vi "Signal Acquisition.vi"(0 "Signals Sampling":T4 {"Sample Mode" items=["Finite Samples"=10178, "Continuous Samples"=10123, "Hardware Timed Single Point"=12522]}, 1 "Pressure Signal":T5 {"Terminal Configuration" items=["Default"=-1, "RSE"=10083, "Differential"=10106, "Pseudodifferential"=12529]; "Scale Type" items=["Volts"=10348, "Custom Scale"=10065]}, 2 "Electrode Signals":T1={"Scale Type"=10348, "Terminal Configuration"=10083, "Scale Name"="", "Range [V]"={"max"=10.0, "min"=-10.0}, "Channel 2 [Potential]"="Dev4/ai2", "Channel 1 [Current]"="Dev4/ai2"} {"Terminal Configuration" items=["Default"=-1, "RSE"=10083, "Differential"=10106, "Pseudodifferential"=12529]; "Scale Type" items=["Volts"=10348, "Custom Scale"=10065]}, 5 "error in":errorcluster, 6 "Indicators":T3, 8 "Filter":refnum<vi>, 10 "Filter Led Indicator":refnum<vi>, 12 "IIR filter specifications":refnum<vi>, 13 "Exit":refnum<vi>) -> (19 "error out":errorcluster)   [LabVIEW 2012, in "Signal Acquisition.lvlib"]
uses:
  Signal Acquisition.lvlib
  <vilib>/DAQmx/read.llb/DAQmx Read (Analog 1D Wfm NChan NSamp).vi
  <vilib>/DAQmx/create/channels.llb/DAQmx Create Channel (AI-Voltage-Basic).vi
  <vilib>/DAQmx/configure/timing.llb/DAQmx Timing (Sample Clock).vi
  <vilib>/measure/madcrms.llb/Basic Averaged DC-RMS for 1 Chan.vi
  <vilib>/measure/maspectr.llb/FFT Power Spectrum and PSD for 1 Chan.vi
  <vilib>/DAQmx/miscellaneous.llb/DAQmx Fill In Error Info.vi
  <vilib>/measure/NI_MAPro.lvlib
  <vilib>/measure/macond.llb/IIR Filter for 1 Chan.vi
panel:
  out "Resistance C":dbl
  out "Current":dbl
  out "Resistance":dbl
  out "Pressure":waveform(dbl)
  out "Current Signal":waveform(dbl)
  out "PSD":cluster{"f0":dbl, "df":dbl, "magnitude":dbl[]} {"magnitude" format="%.2p"; "f0" format="%0.2p"; "df" format="%0.2p"}
  out "Filter":bool
  out "Filter Param":T2
  out "Exit":bool
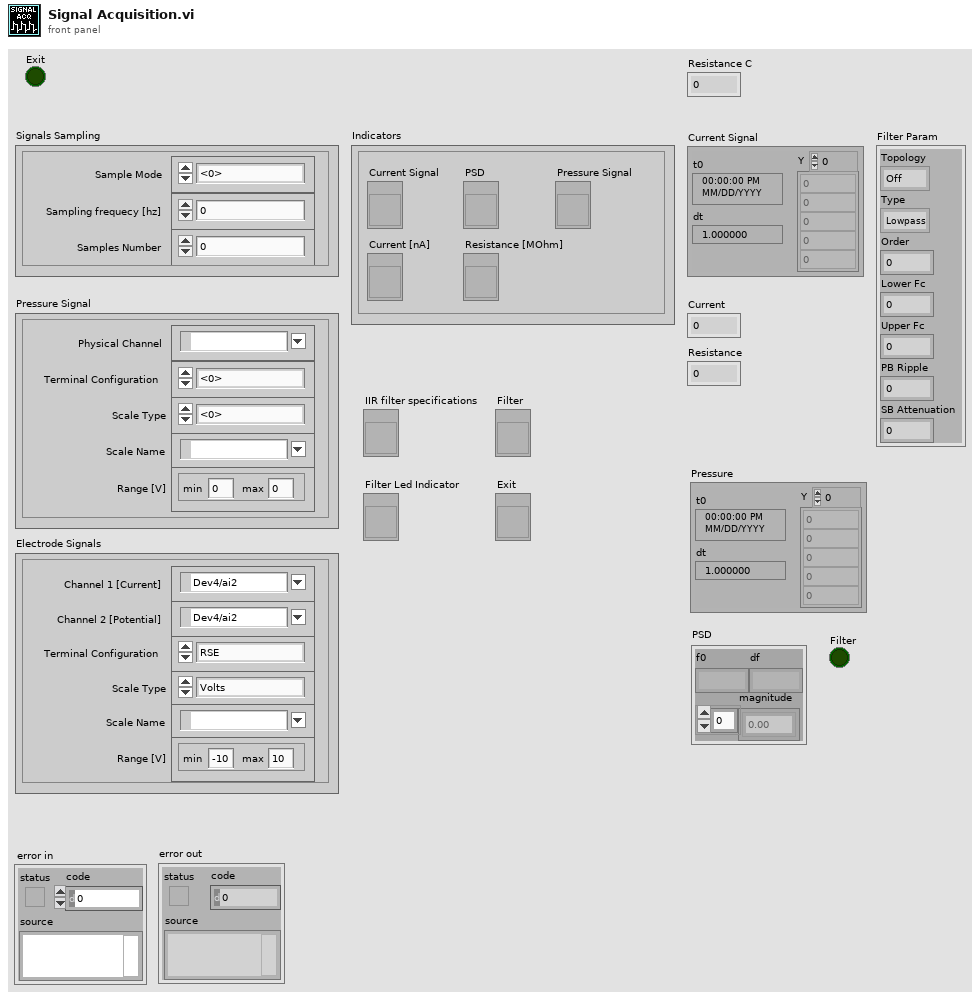
[diagram p1: front panel]
types:
  T1 = cluster{"Scale Type":i32, "Terminal Configuration":i32, "Scale Name":tag, "Range [V]":cluster{"max":dbl, "min":dbl}, "Channel 2 [Potential]":tag, "Channel 1 [Current]":tag}
  T2 = cluster{"Topology":enum16{"Off", "Butterworth", "Chebyshev", "Inverse Chebyshev", "Elliptic", "Bessel"}, "Type":enum16{"Lowpass", "Highpass", "Bandpass", "Bandstop"}, "Order":i32, "Lower Fc":dbl, "Upper Fc":dbl, "PB Ripple":dbl, "SB Attenuation":dbl}
  T3 = cluster{"Current Signal":refnum<vi>, "PSD":refnum<vi>, "Pressure Signal":refnum<vi>, "Current [nA]":refnum<vi>, "Resistance [MOhm]":refnum<vi>}
  T4 = cluster{"Sample Mode":i32, "Sampling frequecy [hz]":dbl, "Samples Number":i32}
  T5 = cluster{"Scale Type":i32, "Terminal Configuration":i32, "Scale Name":tag, "Range [V]":cluster{"max":dbl, "min":dbl}, "Physical Channel":tag}
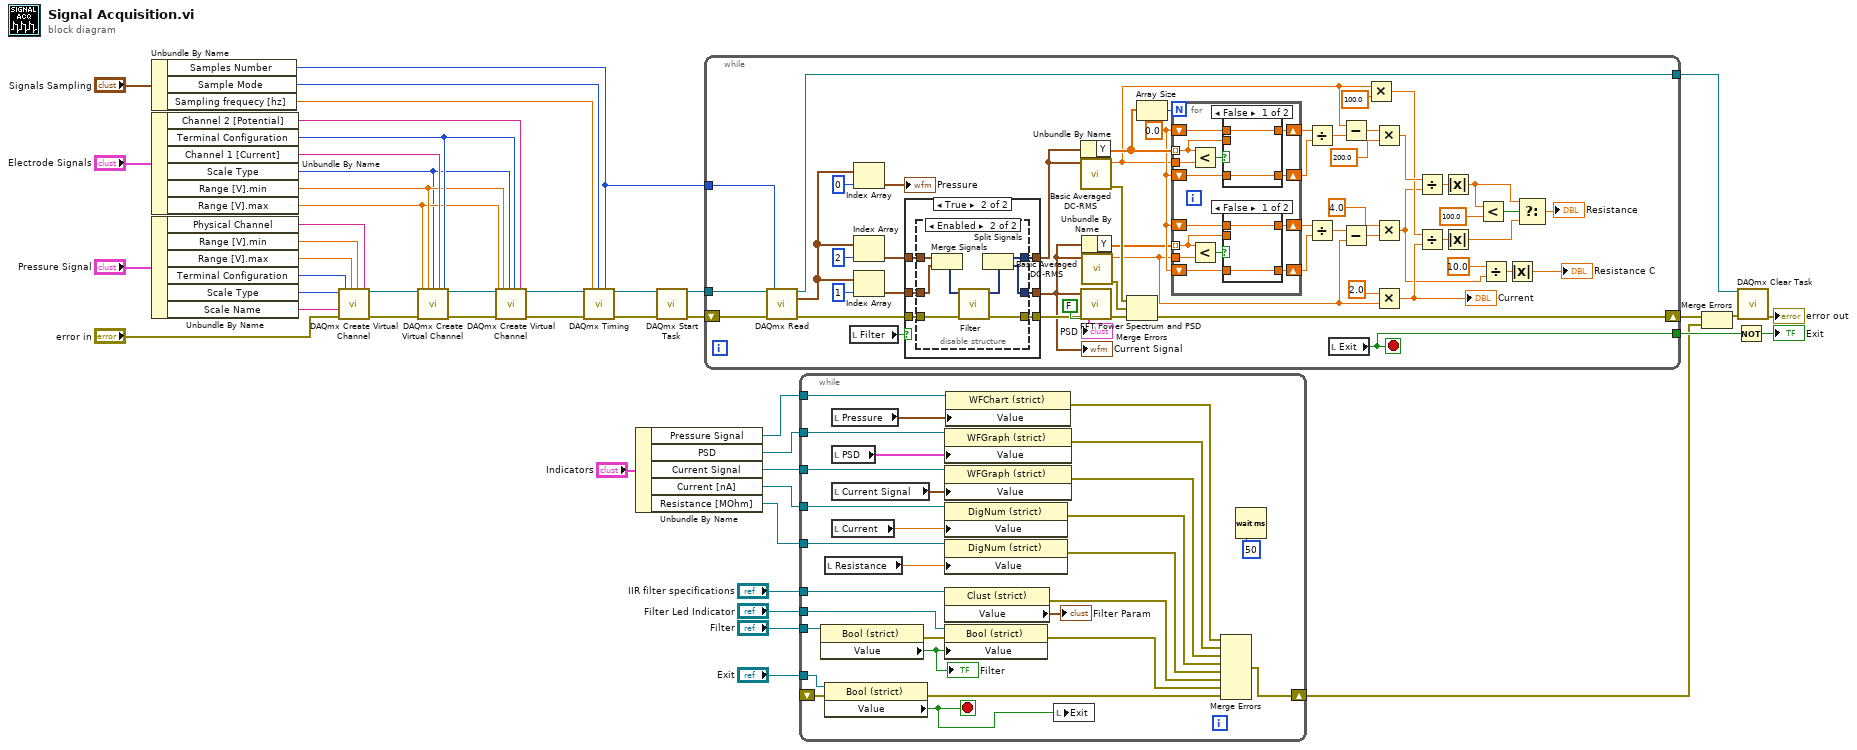
[diagram p0: block diagram]
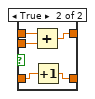
[diagram p2: hidden frame]
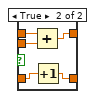
[diagram p3: hidden frame]
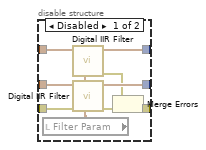
[diagram p5: hidden frame]
diagram:
  n1 = Unbundle By Name("Signals Sampling") -> ("Samples Number"=w26:i32, "Sample Mode"=w25:i32, "Sampling frequecy [hz]"=w24:dbl)
  n2 = Unbundle By Name("Electrode Signals") -> ("Channel 2 [Potential]"=w10:tag, "Terminal Configuration"=w9:i32, "Channel 1 [Current]"=w43:tag, "Scale Type"=w6:i32, "Range [V].min"=w8:dbl, "Range [V].max"=w7:dbl)
  n3 = Unbundle By Name("Pressure Signal") -> ("Physical Channel"=w36:tag, "Range [V].min"=w35:dbl, "Range [V].max"=w34:dbl, "Terminal Configuration"=w33:i32, "Scale Type"=w32:i32, "Scale Name"=w31:tag)
  n4 = call-poly <vilib>:"DAQmx Create Virtual Channel.vi"("maximum value"=w34, "minimum value"=w35, "input terminal configuration"=w33, "physical channels"=w36, "units"=w32, "error in"="error in", "custom scale name"=w31) -> ("task out"=w30:refnum<k21>, "error out"=w29:errorcluster)  [unwired: 7 in]
  n5 = call-poly <vilib>:"DAQmx Create Virtual Channel.vi"("task in"=w30, "maximum value"=w7, "minimum value"=w8, "input terminal configuration"=w9, "physical channels"=w43, "units"=w6, "error in"=w29) -> ("task out"=w11:refnum<k21>, "error out"=w12:errorcluster)  [unwired: 7 in]
  n6 = call-poly <vilib>:"DAQmx Create Virtual Channel.vi"("task in"=w11, "maximum value"=w7, "minimum value"=w8, "input terminal configuration"=w9, "physical channels"=w10, "units"=w6, "error in"=w12) -> ("task out"=w4:refnum<k21>, "error out"=w5:errorcluster)  [unwired: 7 in]
  n7 = call-poly <vilib>:"DAQmx Timing.vi"("task/channels in"=w4, "sample mode"=w25, "samples per channel"=w26, "rate"=w24, "error in"=w5) -> ("task out"=w41:refnum<k21>, "error out"=w42:errorcluster)  [unwired: 9 in]
  n8 = Unbundle By Name("Indicators") -> ("Pressure Signal"=w14:refnum<vi>, "PSD"=w3:refnum<vi>, "Current Signal"=w18:refnum<vi>, "Current [nA]"=w2:refnum<vi>, "Resistance [MOhm]"=w1:refnum<vi>)
  n9 = call <vilib>:"DAQmx Start Task.vi"("task/channels in"=w41, "error in"=w42) -> ("task out"=w39:refnum<k21>, "error out"=w40:errorcluster)  [unwired: 12 out]
  n10 = while {
    tunnel: w39 -> [w101]
    tunnel: w26 -> [w99]
    tunnel: [w98] -> w44
    shift-right: [w66] -> w16
    shift-left: w40 -> [w100]
    tunnel: [w97] -> w45
    stop <- w97 stop-if-true
    w72 = 0.0
    n11 = call-poly <vilib>:"DAQmx Read.vi"("task/channels in"=w101, "number of samples per channel"=w99, "error in"=w100) -> ("task out"=w98:refnum<k21>, "data"=w87:waveform(dbl)[], "error out"=w92:errorcluster)  [unwired: 10 in]
    n12 = local read "Filter"() -> (w91:bool)
    n13 = Index Array(array=w87, index=0) -> (element=→"Pressure":waveform(dbl))
    n14 = Index Array(array=w87, index=2) -> (element=w85:waveform(dbl))
    n15 = Index Array(array=w87, index=1) -> (element=w86:waveform(dbl))
    n16 = case shown="True" w91 {
      tunnel: w86 -> [w130 w138]
      tunnel: [w130 w137] -> w76
      tunnel: w92 -> [w132 w136]
      tunnel: [w132 w133] -> w93
      tunnel: w85 -> [w131 w135]
      tunnel: [w131 w134] -> w61
      frame False {
      }
      frame True {
        n17 = disable-structure shown="Enabled" {
          disable-tunnel: w138 -> [w147 w151]
          disable-tunnel: [w146 w148] -> w137
          disable-tunnel: w136 -> [w145 w155]
          disable-tunnel: w135 -> [w144 w152]
          disable-tunnel: [w142 w149] -> w134
          disable-tunnel: [w140 w154] -> w133
          frame Disabled {
            n18 = local read "Filter Param"() -> (w143:T2)
            n19 = call-poly <vilib>:"Digital IIR Filter.vi"("IIR filter specifications"=w143, "signal in"=w144) -> ("error out"=w139:errorcluster, "signal out"=w142:waveform(dbl))  [unwired: 7 in, 1 out]
            n20 = call-poly <vilib>:"Digital IIR Filter.vi"("IIR filter specifications"=w143, "error in (no error)"=w145, "signal in"=w147) -> ("error out"=w141:errorcluster, "signal out"=w146:waveform(dbl))  [unwired: 6 in, 1 out]
            n21 = Merge Errors(w139, w141) -> (w140:errorcluster)
          }
          frame Enabled {
            n22 = Merge Signals(w152, w151) -> (w150:dynamicdata)
            n23 = call "Filter"("error in (no error)"=w155, "Signal"=w150) -> ("error out"=w154:errorcluster, "Filtered Signal"=w153:dynamicdata)  [unwired: 8 in]
            n24 = Split Signals(w153) -> (w149:dynamicdata, w148:dynamicdata)  [unwired: 2 in]
          }
        }
      }
    }
    "Current Signal" <- w76
    n25 = Unbundle By Name(w61) -> ("Y"=w80:dbl[])
    n26 = call-poly <vilib>:"Basic Averaged DC-RMS.vi"("signal in"=w61) -> ("error out"=w68:errorcluster, "DC value"=w58:dbl)  [unwired: 7 in, 2 out]
    n27 = call-poly <vilib>:"FFT Power Spectrum and PSD.vi"("error in (no error)"=w93, "dB On (F)"=FALSE, "time signal"=w76) -> ("error out"=w70:errorcluster, "Power Spectrum / PSD"=→"PSD":cluster{"f0":dbl, "df":dbl, "magnitude":dbl[]})  [unwired: 5 in, 2 out]
    n28 = Unbundle By Name(w76) -> ("Y"=w67:dbl[])
    n29 = call-poly <vilib>:"Basic Averaged DC-RMS.vi"("signal in"=w76) -> ("error out"=w69:errorcluster, "DC value"=w62:dbl)  [unwired: 7 in, 2 out]
    n30 = Merge Errors(w68, w69, w70) -> (w66:errorcluster)
    n31 = Array Size(array=w80) -> (size(s)=w77:i32)
    n32 = for {
      N: w77 -> [_]
      tunnel: w80 -> [w111] mode=indexing
      tunnel: w58 -> [w115]
      shift-right: [w112] -> w78
      shift-left: w72 -> [w113]
      shift-right: [w109] -> w79
      shift-left: w72 -> [w110]
      tunnel: w67 -> [w106] mode=indexing
      tunnel: w62 -> [w102]
      shift-right: [w105] -> w74
      shift-left: w72 -> [w104]
      shift-right: [w108] -> w73
      shift-left: w72 -> [w107]
      n33 = Less?(x=w111, y=w115) -> (x < y?=w114:bool)
      n34 = Less?(x=w106, y=w102) -> (x < y?=w103:bool)
      n35 = case shown="False" w114 {
        tunnel: w113 -> [w124 w129]
        tunnel: [w124 w128] -> w112
        tunnel: w111 -> [_ w125]
        tunnel: w110 -> [w123 w127]
        tunnel: [w123 w126] -> w109
        frame False {
        }
        frame True {
          n36 = Add(x=w129, y=w125) -> (x+y=w128:dbl)
          n37 = Increment(x=w127) -> (x+1=w126:dbl)
        }
      }
      n38 = case shown="False" w103 {
        tunnel: w104 -> [w117 w122]
        tunnel: [w117 w121] -> w105
        tunnel: w106 -> [_ w118]
        tunnel: w107 -> [w116 w120]
        tunnel: [w116 w119] -> w108
        frame False {
        }
        frame True {
          n39 = Add(x=w122, y=w118) -> (x+y=w121:dbl)
          n40 = Increment(x=w120) -> (x+1=w119:dbl)
        }
      }
    }
    n41 = Divide(x=w78, y=w79) -> (x/y=w75:dbl)
    n42 = Divide(x=w74, y=w73) -> (x/y=w71:dbl)
    n43 = local read "Exit"() -> (w97:bool)
    n44 = Subtract(x=w58, y=w75) -> (x-y=w65:dbl)
    n45 = Subtract(x=w71, y=w62) -> (x-y=w64:dbl)
    n46 = Multiply(x=w58, y=100.0) -> (x*y=w56:dbl)
    n47 = Multiply(x=w65, y=200.0 ("x")) -> (x*y=w84:dbl)
    n48 = Multiply(x=4.0, y=w64) -> (x*y=w48:dbl)
    n49 = Multiply(x=2.0, y=w62) -> (x*y=w59:dbl)
    "Current" <- w59
    n50 = Divide(x=w84, y=w48) -> (x/y=w63:dbl)
    n51 = Divide(x=w56, y=w59) -> (x/y=w60:dbl)
    n52 = Absolute Value(x=w63) -> (abs(x)=w53:dbl)
    n53 = Absolute Value(x=w60) -> (abs(x)=w52:dbl)
    n54 = Less?(x=w53, y=100.0) -> (x < y?=w47:bool)
    n55 = Divide(x=10.0, y=w48) -> (x/y=w51:dbl)
    n56 = Absolute Value(x=w51) -> (abs(x)=→"Resistance C":dbl)
    n57 = Select(t=w53, s=w47, f=w52) -> (s? t:f=→"Resistance":dbl)
  }
  n58 = while {
    tunnel: "Filter Led Indicator" -> [w183]
    tunnel: "Filter" -> [w182]
    tunnel: "Exit" -> [w180]
    tunnel: w3 -> [w178]
    tunnel: w18 -> [w177]
    tunnel: "IIR filter specifications" -> [w175]
    shift-right: [w169] -> w17
    shift-left: _ -> [w170]
    tunnel: w14 -> [w167]
    tunnel: w2 -> [w164]
    tunnel: w1 -> [w158]
    stop <- w168 stop-if-true
    n59 = property class="Bool (strict)"(reference=w182) -> (error out=w174:errorcluster, "Value"=w181:bool)  [unwired: 1 in, 1 out]
    "Filter" <- w181
    n60 = local read "Resistance"() -> (w156:dbl)
    n61 = property class="Bool (strict)"(reference=w180, error in=w170) -> (error out=w173:errorcluster, "Value"=w168:bool)  [unwired: 1 out]
    n62 = local read "Pressure"() -> (w166:waveform(dbl))
    n63 = local read "PSD"() -> (w184:cluster{"f0":dbl, "df":dbl, "magnitude":dbl[]})
    n64 = local read "Current Signal"() -> (w165:waveform(dbl))
    n65 = local read "Current"() -> (w157:dbl)
    n66 = property class="WFGraph (strict)"(reference=w178, "Value"=w184) -> (error out=w162:errorcluster)  [unwired: 1 in, 1 out]
    n67 = property class="WFGraph (strict)"(reference=w177, "Value"=w165) -> (error out=w161:errorcluster)  [unwired: 1 in, 1 out]
    n68 = property class="DigNum (strict)"(reference=w164, "Value"=w157) -> (error out=w160:errorcluster)  [unwired: 1 in, 1 out]
    n69 = property class="DigNum (strict)"(reference=w158, "Value"=w156) -> (error out=w159:errorcluster)  [unwired: 1 in, 1 out]
    n70 = property class="Clust (strict)"(reference=w175) -> (error out=w171:errorcluster, "Value"=→"Filter Param":T2)  [unwired: 1 in, 1 out]
    n71 = property class="Bool (strict)"(reference=w183, error in=w174, "Value"=w181) -> (error out=w172:errorcluster)  [unwired: 1 out]
    n72 = property class="WFChart (strict)"(reference=w167, "Value"=w166) -> (error out=w163:errorcluster)  [unwired: 1 in, 1 out]
    n73 = local write "Exit"(w168) -> ()
    n74 = Merge Errors(w163, w162, w161, w160, w159, w171, w172, w173) -> (w169:errorcluster)
    n75 = Wait (ms)(milliseconds to wait=u32 50) -> ()  [unwired: 1 out]
  }
  n76 = Merge Errors(w16, w17) -> (w15:errorcluster)
  n77 = Not(x=w45) -> (.not. x?=→"Exit":bool)
  n78 = call <vilib>:"DAQmx Clear Task.vi"("task in"=w44, "error in"=w15) -> ("error out"=→"error out":errorcluster)  [unwired: 13 in]
